vi "Create 0mqPorts.vi"(9 "level":u32 caption="level (0, 1, 2, or 3)" max=3, 10 "sysName":string) -> (0 "repPort":string, 1 "reqPort":string, 2 "subPort":string, 3 "pubPort":string, 4 "repPort":u16, 5 "subPort":u16, 6 "reqPort":u16, 7 "pubPort":u16)   [LabVIEW 2018]
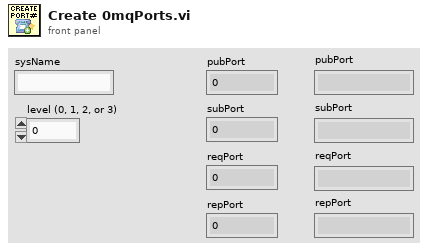
[diagram p1: front panel]
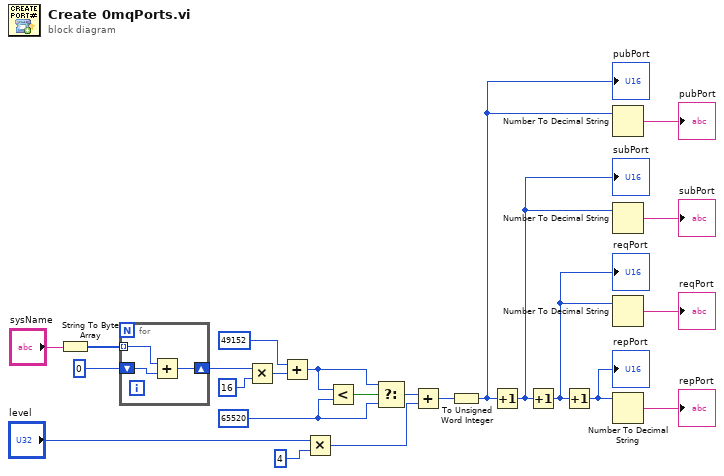
[diagram p0: block diagram]
diagram:
  w10 = u32 65520
  n1 = String To Byte Array(string="sysName") -> (unsigned byte array=w22:u8[])
  n2 = for {
    tunnel: w22 -> [w25] mode=indexing
    shift-right: [w26] -> w20
    shift-left: u32 0 -> [w24]
    n3 = Add(x=w25, y=w24) -> (x+y=w26:u32)
  }
  n4 = Multiply(x=w20, y=u32 16) -> (x*y=w17:u32)
  n5 = Add(x=u32 49152, y=w17) -> (x+y=w9:u32)
  n6 = Multiply(x="level", y=u32 4) -> (x*y=w14:u32)
  n7 = Less?(x=w9, y=w10) -> (x < y?=w11:bool)
  n8 = Select(t=w9, s=w11, f=w10) -> (s? t:f=w12:u32)
  n9 = Add(x=w12, y=w14) -> (x+y=w13:u32)
  n10 = To Unsigned Word Integer(number=w13) -> (unsigned 16bit integer=w8:u16)
  "pubPort" <- w8
  n11 = Increment(x=w8) -> (x+1=w6:u16)
  "subPort" <- w6
  n12 = Increment(x=w6) -> (x+1=w4:u16)
  "reqPort" <- w4
  n13 = Increment(x=w4) -> (x+1=w2:u16)
  "repPort" <- w2
  n14 = Number To Decimal String(number=w8) -> (decimal integer string=→"pubPort":string)  [unwired: 1 in]
  n15 = Number To Decimal String(number=w6) -> (decimal integer string=→"subPort":string)  [unwired: 1 in]
  n16 = Number To Decimal String(number=w4) -> (decimal integer string=→"reqPort":string)  [unwired: 1 in]
  n17 = Number To Decimal String(number=w2) -> (decimal integer string=→"repPort":string)  [unwired: 1 in]
